vi "FABR-Init Analysis.vi"(0 "Params":T3 {"Response"."Window (ms)" format="%.2f"; "Stimulus"."Start (kHz)" step=5.0; "Stimulus"."Start (dB)" step=5}, 5 "Runtime in":T7, 7 "SCL in":T1[](array[typedef]), 11 "error in (no error)":errorcluster) -> (4 "Analysis":T2, 6 "Runtime out":T7, 8 "SCL out":T1[](array[typedef]), 15 "error out":errorcluster)   [LabVIEW 2020]
uses:
  Typedefs/FABR-Runtime Data.ctl
  Typedefs/FABR-Parameters.ctl
  Typedefs/FABR-Stimulus.ctl
  Typedefs/FABR-Response.ctl
  Typedefs/FABR-Hidden Params.ctl
  Typedefs/FABR-Analysis State.ctl
  Typedefs/FABR-Stimulus Condition.ctl
panel:
  # "Freq X Level X Time"
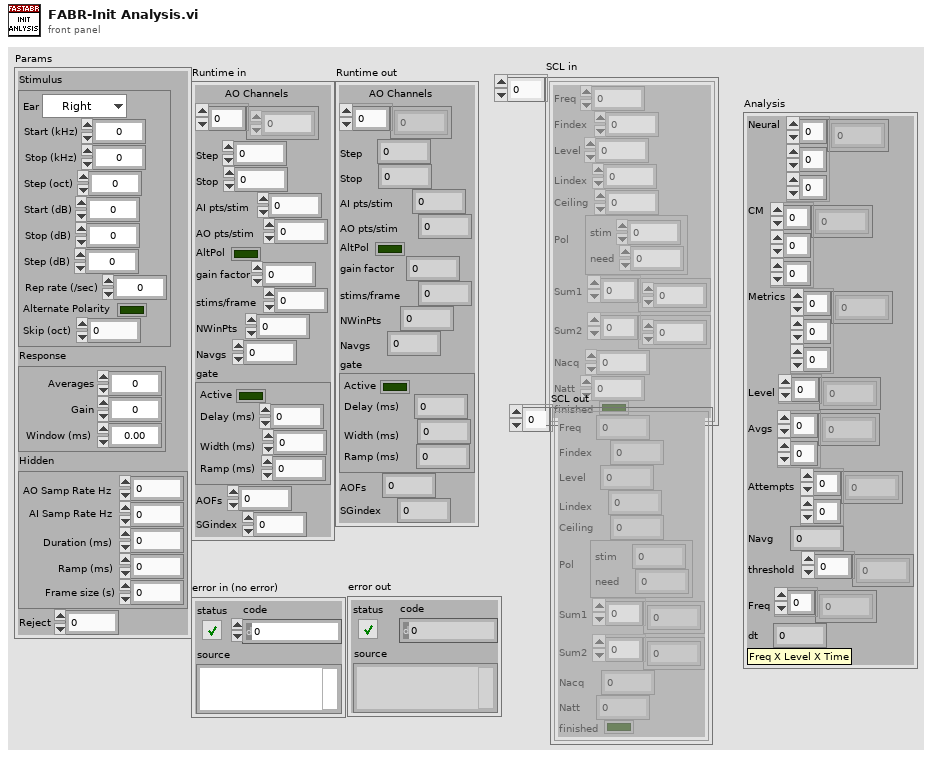
[diagram p1: front panel]
types:
  T1 = typedef "FABR-Stimulus Condition.ctl" = cluster{"Freq":dbl, "Findex":i32, "Level":dbl, "Lindex":i32, "Ceiling":dbl, "Pol":cluster{"stim":i32, "need":i32}, "Sum1":dbl[], "Sum2":dbl[], "Nacq":i32, "Natt":i32, "finished":bool}
  T2 = typedef "FABR-Analysis State.ctl" = cluster{"Neural":dbl[][][], "CM":dbl[][][], "Metrics":dbl[][][], "Level":dbl[], "Avgs":i32[][], "Attempts":i32[][], "Navg":i32, "threshold":dbl[], "Freq":dbl[], "dt":dbl}
  T3 = typedef "FABR-Parameters.ctl" = cluster{"Stimulus":T4, "Response":T5, "Hidden":T6, "Reject":dbl}
  T4 = typedef "FABR-Stimulus.ctl" = cluster{"Ear":enum16{"Right", "Left"}, "Start (kHz)":dbl, "Stop (kHz)":dbl, "Step (oct)":dbl, "Start (dB)":i32, "Stop (dB)":i32, "Step (dB)":i32, "Rep rate (/sec)":dbl, "Alternate Polarity":bool, "Skip (oct)":dbl}
  T5 = typedef "FABR-Response.ctl" = cluster{"Gain":dbl, "Averages":i32, "Window (ms)":sgl}
  T6 = typedef "FABR-Hidden Params.ctl" = cluster{"AI Samp Rate Hz":dbl, "AO Samp Rate Hz":dbl, "Duration (ms)":dbl, "Ramp (ms)":dbl, "Frame size (s)":dbl}
  T7 = typedef "FABR-Runtime Data.ctl" = cluster{"AO Channels":i32[], "Step":dbl, "Stop":i32, "AI pts/stim":i32, "AO pts/stim":i32, "AltPol":bool, "gain factor":dbl, "stims/frame":i32, "NWinPts":i32, "Navgs":i32, "gate":cluster{"Active":bool, "Delay (ms)":dbl, "Width (ms)":dbl, "Ramp (ms)":dbl}, "AOFs":dbl, "SGindex":i32}
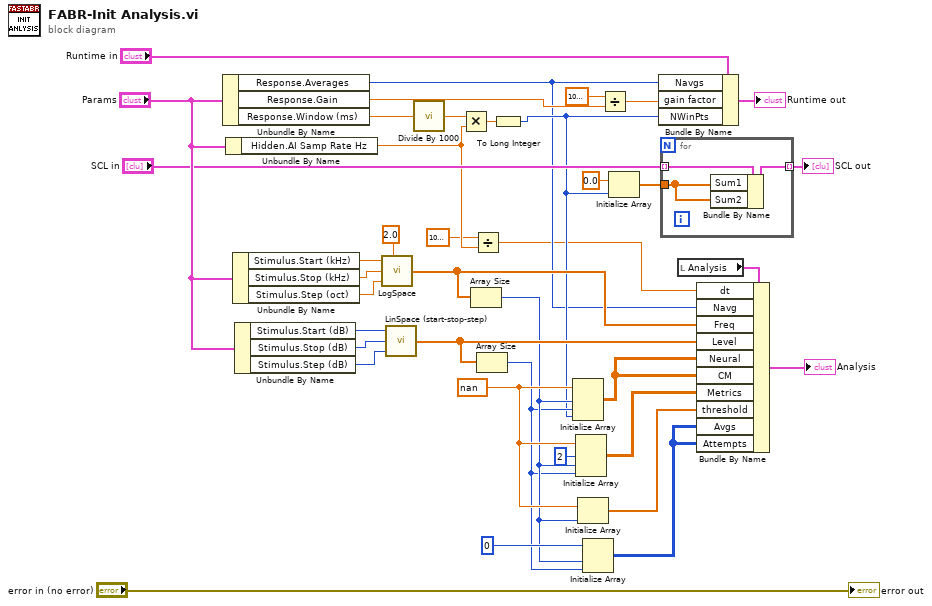
[diagram p0: block diagram]
diagram:
  w18 = nan ("element")
  n1 = Unbundle By Name("Params") -> ("Response.Averages"=w4:i32, "Response.Gain"=w10:dbl, "Response.Window (ms)"=w35:sgl)
  n2 = Unbundle By Name("Params") -> ("Hidden.AI Samp Rate Hz"=w3:dbl)
  n3 = Unbundle By Name("Params") -> ("Stimulus.Start (kHz)"=w28:dbl, "Stimulus.Stop (kHz)"=w27:dbl, "Stimulus.Step (oct)"=w25:dbl)
  n4 = Unbundle By Name("Params") -> ("Stimulus.Start (dB)"=w37:i32, "Stimulus.Stop (dB)"=w38:i32, "Stimulus.Step (dB)"=w39:i32)
  n5 = call "LogSpace.vi"("Start"=w28, "Base"=2.0, "Stop"=w27, "Step"=w25) -> ("Array"=w24:dbl[])  [unwired: 2 in, 1 out]
  n6 = call "LinSpace (start-stop-step).vi"("Step"=w39, "Stop"=w38, "Start"=w37) -> ("Array"=w23:dbl[])  [unwired: 1 in, 1 out]
  n7 = call "Divide By 1000.vi"("X"=w35) -> ("X/1000"=w36:dbl)
  n8 = Multiply(x=w36, y=w3) -> (x*y=w34:dbl)
  n9 = Array Size(array=w24) -> (size(s)=w15:i32)
  n10 = Divide(x=1000000.0, y=w3) -> (x/y=w2:dbl)
  n11 = Array Size(array=w23) -> (size(s)=w14:i32)
  n12 = To Long Integer(number=w34) -> (32bit integer=w7:i32)
  n13 = Initialize Array(w18, w15, w14, w7) -> (w21:dbl[][][])
  n14 = Initialize Array(w18, 2 ("dimension size"), w15, w14) -> (w19:dbl[][][])
  n15 = Initialize Array(w18, w15) -> (w17:dbl[])
  n16 = Initialize Array(0, w15, w14) -> (w13:i32[][])
  n17 = Divide(x=1000000.0, y=w10) -> (x/y=w12:dbl)
  n18 = Initialize Array(0.0 ("element"), w7) -> (w5:dbl[])
  n19 = Bundle By Name(cluster="Runtime in", "Navgs"=w4, "gain factor"=w12, "NWinPts"=w7) -> (→"Runtime out":T7)
  n20 = for {
    tunnel: "SCL in" -> [w42] mode=indexing
    tunnel: [w41] -> w8 mode=indexing
    tunnel: w5 -> [w40]
    n21 = Bundle By Name(cluster=w42, "Sum1"=w40, "Sum2"=w40) -> (w41:T1)
  }
  "SCL out" <- w8
  n22 = local read "Analysis"() -> (w33:T2)
  n23 = Bundle By Name(cluster=w33, "dt"=w2, "Navg"=w4, "Freq"=w24, "Level"=w23, "Neural"=w21, "CM"=w21, "Metrics"=w19, "threshold"=w17, "Avgs"=w13, "Attempts"=w13) -> (→"Analysis":T2)
  "error out" <- "error in (no error)"
